vi "Legend Palette.vi"(4 "Active Plot":i32, 6 "Control Ref Queue":T4, 9 "Window Bounds":T5, 10 "Multiplot Representation In":T1, 11 "2D Feather.lvclass in":refnum<class "2D Feather.lvclass">) -> (1 "Cancel?":bool, 2 "Multiplot Representation Out":T1, 3 "2D Feather.lvclass out":refnum<class "2D Feather.lvclass">)   [LabVIEW 2017, in "2D Feather.lvclass"]
uses:
  <vilib>/Math Plots/2D Math Plots/2D Feather/2D Feather/2D Feather.lvclass
  e:/builds/penguin/labview/branches/2017/dev/dist/vi.lib/Math Plots/2D Math Plots/2D Plot/2D Plot/2D Plot.lvclass
  <vilib>/Math Plots/2D Math Plots/2D Plot/Action String/2DMathPlot Ctrl Act Queue.ctl
  <vilib>/Math Plots/2D Math Plots/2D Plot/Action String/2DMathPlot Ctrl Act Cluster.ctl
  <vilib>/Math Plots/2D Math Plots/2D Plot/Action String/2DMathPlot State Class.ctl
  <vilib>/Math Plots/2D Math Plots/2D Plot/2D Plot/Typedef/Multiplot Representation.ctl
  <vilib>/Math Plots/2D Math Plots/2D Plot/2D Plot/Typedef/Plot Representation.ctl
  <vilib>/Math Plots/2D Math Plots/2D Plot/2D Plot/Typedef/Range Cluster.ctl
  <vilib>/Utility/miscctls.llb/LVRectTypeDef.ctl
  <vilib>/Math Plots/2D Math Plots/2D Feather/2D Feather/2D Feather.lvclass/2D Feather.ctl
  <vilib>/Math Plots/2D Math Plots/2D Plot/2D Plot/2D Plot.lvclass
panel:
  in  "Tab Control":enum32{"Plot Property", "Input & Output"}(tab)
  in  "Line Width":u16(ring) caption="Line width"
  in  "Line Style":u16(ring) caption="Line style"
  in  "OK":bool
  in  "Cancel":bool
  in  "Feather Size":dbl caption="Feather size"
  in  "Feather Color":u32(colorbox)
  # "Line style"
  # "Line width"
  # "Feather size"
  # "Feather color"
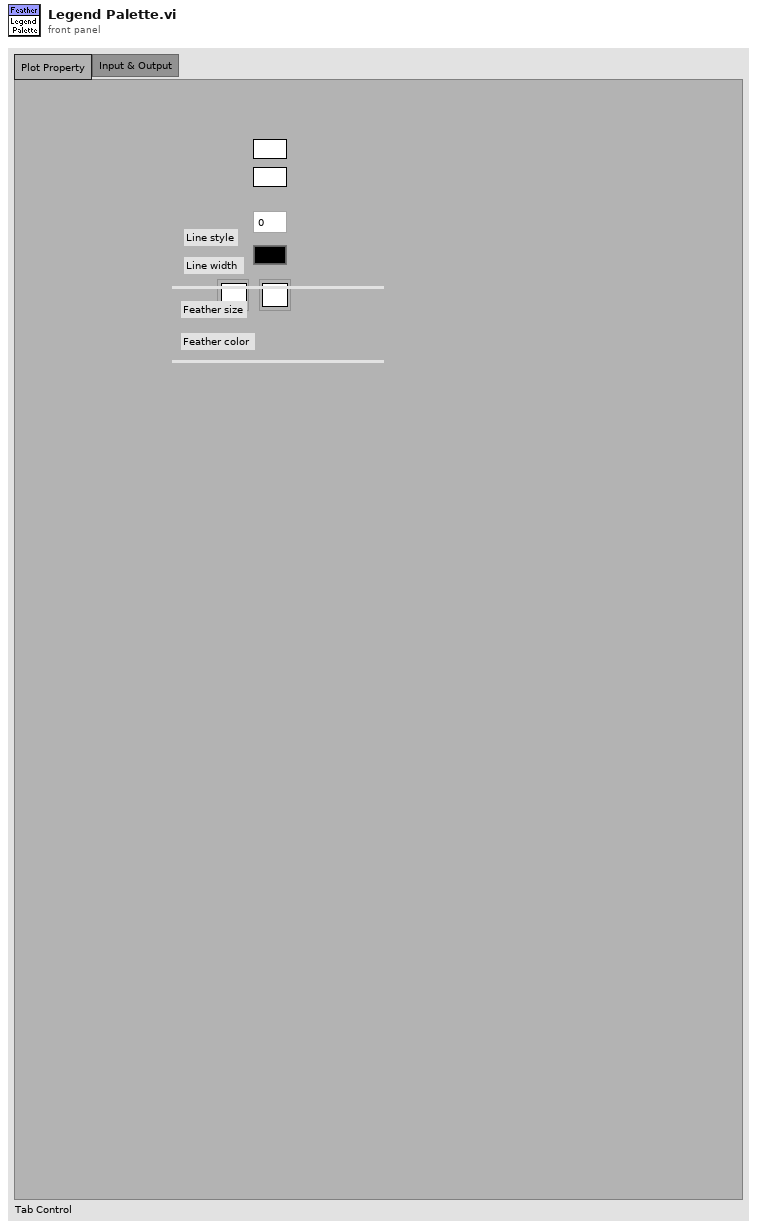
[diagram p1: front panel]
types:
  T1 = typedef "2D Plot.lvclass/Multiplot Representation.ctl" = cluster{"Plot Representation Array":T2[], "Max Range":T3}
  T2 = typedef "2D Plot.lvclass/Plot Representation.ctl" = cluster{"Plot Range":T3, "Vertex Cluster":cluster{"Vertex X Array":dbl[], "Vertex Y Array":dbl[]}, "Base Cluster":cluster{"Base X Array":dbl[], "Base Y Array":dbl[]}}
  T3 = typedef "2D Plot.lvclass/Range Cluster.ctl" = cluster{"X Range":cluster{"Max X":dbl, "Min X":dbl}, "Y Range":cluster{"Max Y":dbl, "Min Y":dbl}}
  T4 = typedef "2DMathPlot Ctrl Act Queue.ctl" = refnum<queue>
  T5 = typedef "LVRectTypeDef.ctl" = cluster{"Left":i16, "Top":i16, "Right":i16, "Bottom":i16}
  T6 = typedef "2DMathPlot Ctrl Act Cluster.ctl" = cluster{"Plot Area Ref":refnum<vi>, "Z Axis Ref":refnum<vi>, "Legend Ref":refnum<vi>, "XControl Ref":refnum<vi>, "Facade Ref":refnum<vi>, "Display State Change Class":T7}
  T7 = typedef "2DMathPlot State Class.ctl" = enum16{"Update All (Undo)", "Update General", "Update Appearance", "Update Format", "Update Scale", "Update Marker", "Update Cursor", "None"}
  T8 = typedef "2D Plot.lvclass/Plot Property Array.ctl" = T9[]
  T9 = typedef "2D Plot.lvclass/Plot Property.ctl" = cluster{"Bar Plot Style":u8, "DigitalLineStyle":u8, "TransitionLocation":u8, "Transition Type":u8, "Fill To":i16, "Fill/Pt. Color":u32, "Label Style":u8, "Line Style":u8, "Line Width":u8, "Plot Color":u32, "Plot Interpolation":u8, "Plot Name":string, "Point Style":u8, "Visible?":bool, "XScaleIdx":u32, "YScaleIdx":u32}
  T10 = typedef "2D Feather.lvclass/2D Feather Property Array.ctl" = T11[]
  T11 = typedef "2D Feather.lvclass/2D Feather Property.ctl" = cluster{"Arrow Size":dbl}
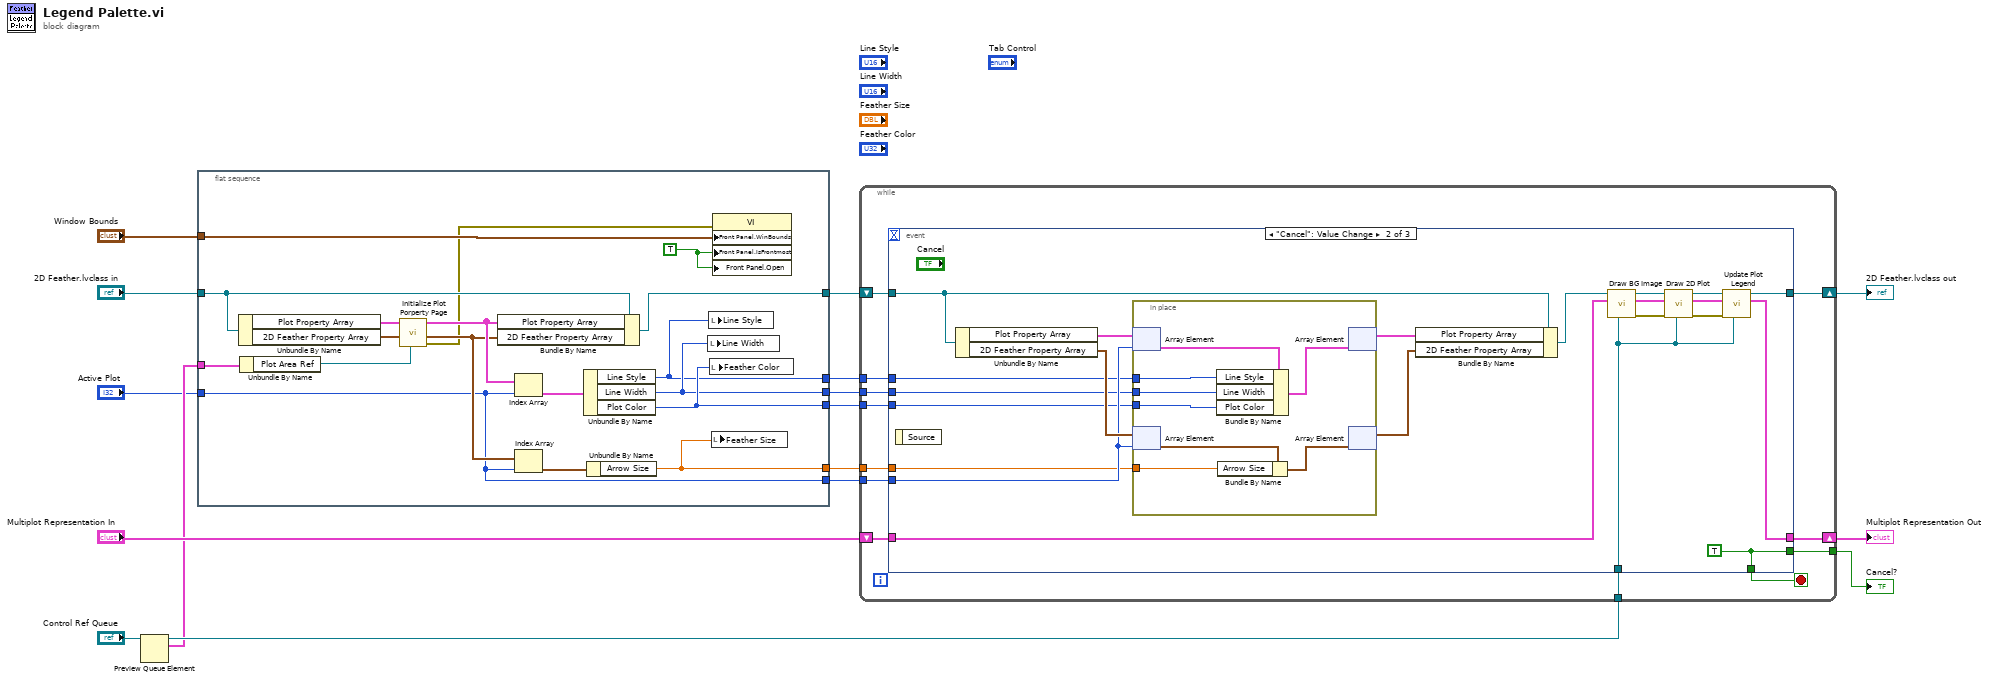
[diagram p0: block diagram]
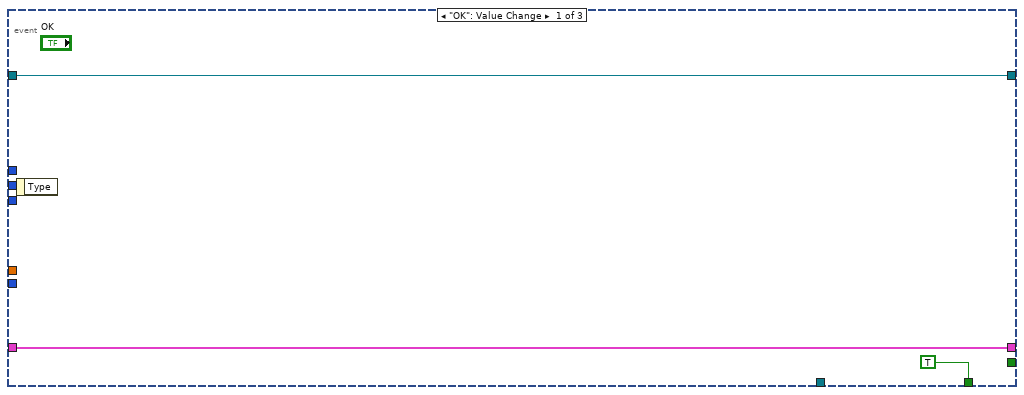
[diagram p2: hidden frame]
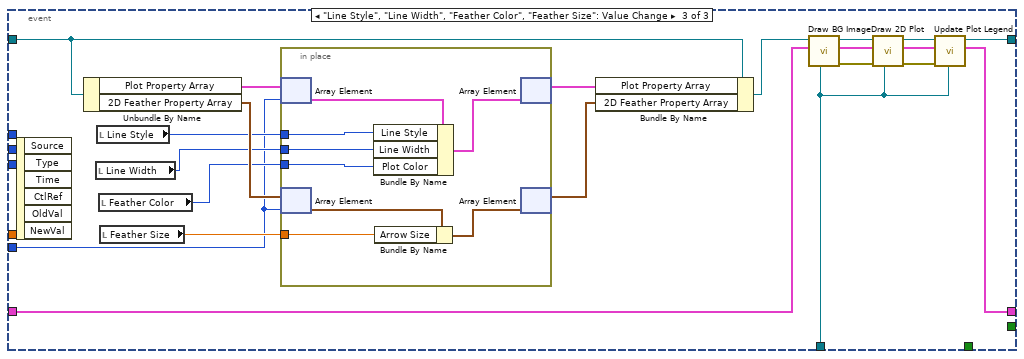
[diagram p3: hidden frame]
diagram:
  n1 = Preview Queue Element(queue="Control Ref Queue") -> (queue out=w10:T4, element=w9:T6)  [unwired: 1 in, 3 out]
  n2 = flat-sequence {
    tunnel: "2D Feather.lvclass in" -> [w26]
    tunnel: [w25] -> w14
    tunnel: [w17] -> w4
    tunnel: w9 -> [w32]
    tunnel: [w30] -> w8
    tunnel: [w29] -> w7
    tunnel: [w28] -> w6
    tunnel: [w27] -> w5
    tunnel: "Window Bounds" -> [w19]
    tunnel: "Active Plot" -> [w17]
    frame #0 {
      w31 = TRUE ("Front Panel Window:Is Frontmost")
      n3 = Unbundle By Name(w26) -> ("Plot Property Array"=w24:T8, "2D Feather Property Array"=w20:T10)
      n4 = Unbundle By Name(w32) -> ("Plot Area Ref"=w22:refnum<vi>)
      n5 = call <vilib>:"Initialize Plot Porperty Page.vi"("Plot Area Ref"=w22, "2D Featherr Array In"=w20, "Plot Property Array In"=w24) -> ("error out"=w18:errorcluster, "2D Feather Array Out"=w21:T10, "Plot Property Array Out"=w23:T8)  [unwired: 2 in, 4 out]
      n6 = Bundle By Name(cluster=w26, "Plot Property Array"=w23, "2D Feather Property Array"=w21) -> (w25:refnum<class "2D Feather.lvclass">)
      n7 = Index Array(array=w23, index=w17) -> (element=w34:T9)
      n8 = Index Array(array=w21, index=w17) -> (element=w33:T11)
      n9 = Unbundle By Name(w34) -> ("Line Style"=w27:u8, "Line Width"=w28:u8, "Plot Color"=w29:u32)
      n10 = Unbundle By Name(w33) -> ("Arrow Size"=w30:dbl)
      n11 = local write "Line Width"(w28) -> ()
      n12 = local write "Line Style"(w27) -> ()
      n13 = local write "Feather Color"(w29) -> ()
      n14 = local write "Feather Size"(w30) -> ()
      n15 = property class="VI"(error in=w18, "Front Panel.WinBounds"=w19, "Front Panel.IsFrontmost"=w31, "Front Panel.Open"=w31) -> ()  [unwired: 1 in, 2 out]
    }
  }
  n16 = while {
    shift-right: [w45] -> w16
    shift-left: w14 -> [w46]
    shift-right: [w43] -> w12
    shift-left: "Multiplot Representation In" -> [w44]
    tunnel: w10 -> [w42]
    tunnel: w4 -> [w41]
    tunnel: w8 -> [w39]
    tunnel: w7 -> [w38]
    tunnel: w6 -> [w37]
    tunnel: w5 -> [w36]
    tunnel: [w35] -> w3
    stop <- w40 stop-if-true
    n17 = event shown="[1] \"Cancel\": Value Change" {
      selector: _ -> [_ _ _]
      dyn-events: _ -> [_ _ _]
      timeout: _ -> [_ _ _]
      tunnel: w46 -> [w49 w66 w98]
      tunnel: [w49 w59 w88] -> w45
      tunnel: w44 -> [w48 w65 w90]
      tunnel: [w48 w58 w87] -> w43
      tunnel: w42 -> [_ w51 w80]
      tunnel: w41 -> [_ w64 w89]
      tunnel: [TRUE w50 _] -> w40
      tunnel: w39 -> [_ w63 _]
      tunnel: w38 -> [_ w62 _]
      tunnel: w37 -> [_ w61 _]
      tunnel: w36 -> [_ w60 _]
      tunnel: [_ w50 _] -> w35
      event "OK": Value Change {
        n18 = event-data() -> ()  [unwired: 2 out]
      }
      event "Cancel": Value Change {
        w50 = TRUE
        n19 = event-data() -> ()  [unwired: 2 out]
        n20 = Unbundle By Name(w66) -> ("Plot Property Array"=w71:T8, "2D Feather Property Array"=w70:T10)
        n21 = in-place {
          in-place-border: w63 -> [w75]
          in-place-border: w60 -> [w74]
          in-place-border: w61 -> [w73]
          in-place-border: w62 -> [w72]
          n22 = in-place-array #1(w71, w64) -> (w79:T9)
          n23 = in-place-array #2(w70, w64) -> (w78:T11)
          n24 = Bundle By Name(cluster=w79, "Line Style"=w74, "Line Width"=w73, "Plot Color"=w72) -> (w76:T9)
          n25 = Bundle By Name(cluster=w78, "Arrow Size"=w75) -> (w77:T11)
          n26 = in-place-array #1(w76) -> (w69:T8)  [unwired: 1 out]
          n27 = in-place-array #2(w77) -> (w68:T10)  [unwired: 1 out]
        }
        n28 = Bundle By Name(cluster=w66, "Plot Property Array"=w69, "2D Feather Property Array"=w68) -> (w67:refnum<class "2D Feather.lvclass">)
        n29 = call-dynamic "Draw BG Image.vi"("Control Ref Queue"=w51, "Multiplot Representation In"=w65, "2D Feather.lvclass in"=w67) -> ("error out"=w57:errorcluster, "Multiplot Representation Out"=w56:T1, "2D Feather.lvclass out"=w55:refnum<class "2D Feather.lvclass">)  [unwired: 1 in, 5 out]
        n30 = call-dynamic "Draw 2D Plot.vi"("Control Ref Queue"=w51, "error in (no error)"=w57, "Multiplot Representation In"=w56, "2D Feather.lvclass in"=w55) -> ("error out"=w52:errorcluster, "Multiplot Representation Out"=w53:T1, "2D Feather.lvclass out"=w54:refnum<class "2D Feather.lvclass">)  [unwired: 5 out]
        n31 = call <vilib>:"Update Plot Legend.vi"("Control Ref Queue"=w51, "error in (no error)"=w52, "Multiplot Representation In"=w53, "2D Plot in"=w54) -> ("Multiplot Representation Out"=w58:T1, "2D Plot out"=w59:refnum<class "2D Feather.lvclass">)  [unwired: 6 out]
      }
      event "Line Style", "Line Width", "Feather Color", "Feather Size": Value Change {
        n32 = event-data() -> ()  [unwired: 7 out]
        n33 = Unbundle By Name(w98) -> ("Plot Property Array"=w100:T8, "2D Feather Property Array"=w99:T10)
        n34 = local read "Line Width"() -> (w93:u16)
        n35 = local read "Line Style"() -> (w94:u16)
        n36 = local read "Feather Color"() -> (w92:u32)
        n37 = local read "Feather Size"() -> (w95:dbl)
        n38 = in-place {
          in-place-border: w95 -> [w104]
          in-place-border: w94 -> [w103]
          in-place-border: w93 -> [w102]
          in-place-border: w92 -> [w101]
          n39 = in-place-array #3(w100, w89) -> (w108:T9)
          n40 = in-place-array #4(w99, w89) -> (w107:T11)
          n41 = Bundle By Name(cluster=w108, "Line Style"=w103, "Line Width"=w102, "Plot Color"=w101) -> (w105:T9)
          n42 = Bundle By Name(cluster=w107, "Arrow Size"=w104) -> (w106:T11)
          n43 = in-place-array #3(w105) -> (w97:T8)  [unwired: 1 out]
          n44 = in-place-array #4(w106) -> (w96:T10)  [unwired: 1 out]
        }
        n45 = Bundle By Name(cluster=w98, "Plot Property Array"=w97, "2D Feather Property Array"=w96) -> (w91:refnum<class "2D Feather.lvclass">)
        n46 = call-dynamic "Draw BG Image.vi"("Control Ref Queue"=w80, "Multiplot Representation In"=w90, "2D Feather.lvclass in"=w91) -> ("error out"=w86:errorcluster, "Multiplot Representation Out"=w85:T1, "2D Feather.lvclass out"=w84:refnum<class "2D Feather.lvclass">)  [unwired: 1 in, 5 out]
        n47 = call-dynamic "Draw 2D Plot.vi"("Control Ref Queue"=w80, "error in (no error)"=w86, "Multiplot Representation In"=w85, "2D Feather.lvclass in"=w84) -> ("error out"=w81:errorcluster, "Multiplot Representation Out"=w82:T1, "2D Feather.lvclass out"=w83:refnum<class "2D Feather.lvclass">)  [unwired: 5 out]
        n48 = call <vilib>:"Update Plot Legend.vi"("Control Ref Queue"=w80, "error in (no error)"=w81, "Multiplot Representation In"=w82, "2D Plot in"=w83) -> ("Multiplot Representation Out"=w87:T1, "2D Plot out"=w88:refnum<class "2D Feather.lvclass">)  [unwired: 6 out]
      }
    }
  }
  "2D Feather.lvclass out" <- w16
  "Multiplot Representation Out" <- w12
  "Cancel?" <- w3
